vi "saveSequence.vi"(0 "object in":refnum<class "Hamamatsu.lvclass">, 2 "folder path":path, 5 "error in (no error)":errorcluster) -> (14 "object out":refnum<class "Hamamatsu.lvclass">, 16 "Timestamps":dbl[](array[numeric]), 17 "Filenames":path[](array[path]), 19 "error out":errorcluster)   [LabVIEW 2021, in "Hamamatsu.lvclass"]
uses:
  Hamamatsu.lvclass
  Hamamatsu.lvclass/Hamamatsu.ctl
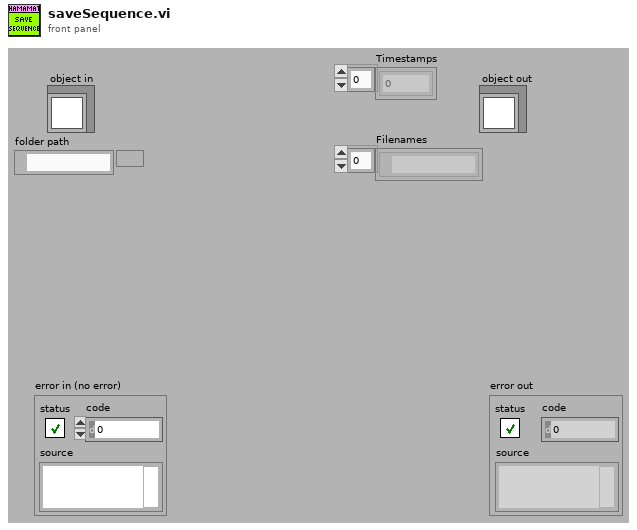
[diagram p1: front panel]
types:
  T1 = typedef "Image Type" = u32
  T2 = typedef "IMAQ Image.ctl" = refnum<image>
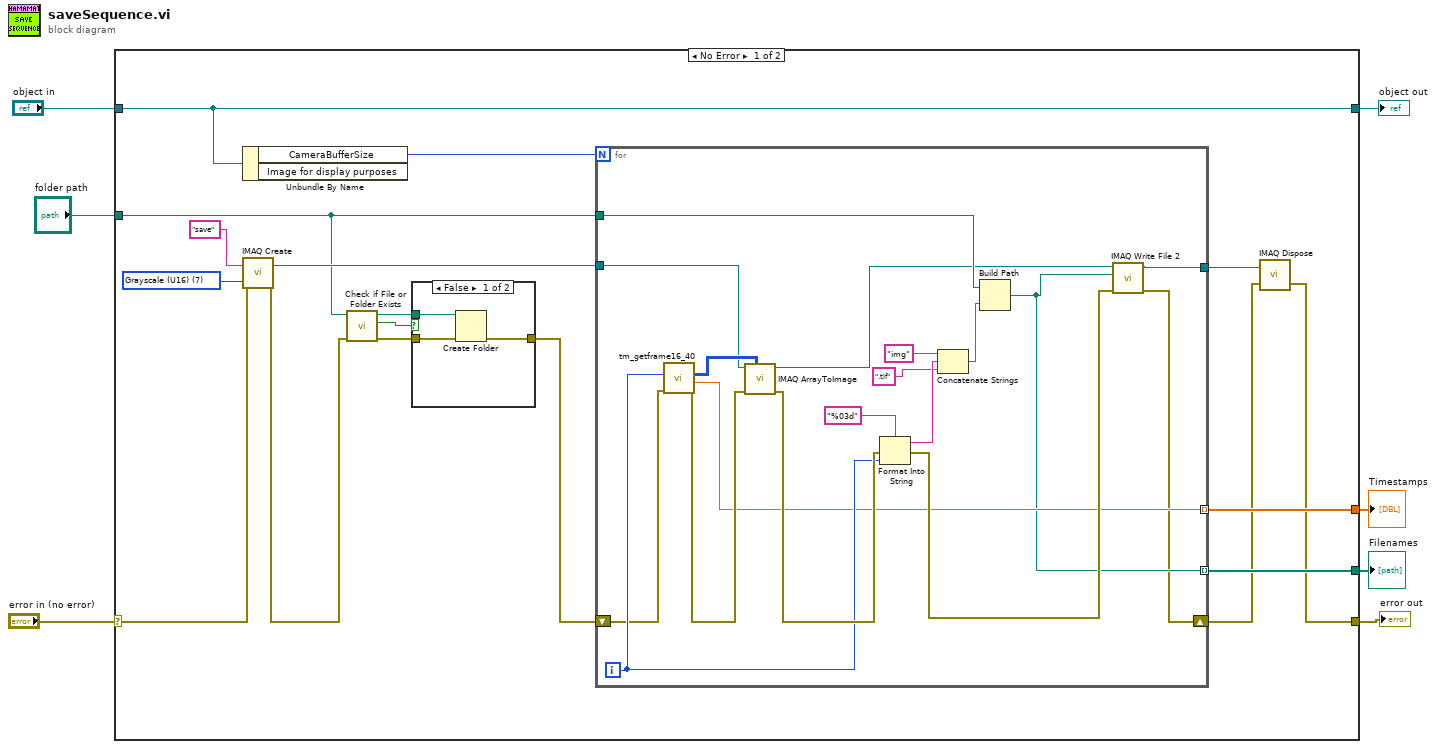
[diagram p0: block diagram]
diagram:
  n1 = case shown="No Error" "error in (no error)" {
    selector: "error in (no error)" -> [w19 w48]
    tunnel: [w14 w48] -> w6
    tunnel: [w24 w47] -> w4
    tunnel: "object in" -> [w24 w47]
    tunnel: "folder path" -> [w13 _]
    tunnel: [w18 _] -> w2
    tunnel: [w17 _] -> w1
    frame No Error {
      w20 = T1 7 items=["Grayscale (U8)", "Grayscale (I16)", "Grayscale (SGL)", "Complex (CSG)", "RGB (U32)", "HSL (U32)", "RGB (U64)", "Grayscale (U16)"] ("Image Type")
      n2 = Unbundle By Name(w24) -> ("CameraBufferSize"=w23:i32)  [unwired: 1 out]
      n3 = call "IMAQ Create"("Image Name"="save", "Image Type"=w20, "error in (no error)"=w19) -> ("New Image"=w21:T2, "error out"=w11:errorcluster)  [unwired: 2 in]
      n4 = call <vilib>:"Check if File or Folder Exists.vi"("error in (no error)"=w11, "path"=w13) -> ("error out"=w9:errorcluster, "file or folder exists?"=w10:bool, "dup path"=w12:path)  [unwired: 7 in]
      n5 = case shown="False" w10 {
        tunnel: w12 -> [w45 _]
        tunnel: w9 -> [w44 w46]
        tunnel: [w43 w46] -> w8
        frame False {
          n6 = Create Folder(path (use dialog)=w45, error in=w44) -> (error out=w43:errorcluster)  [unwired: 1 in, 2 out]
        }
        frame True {
        }
      }
      n7 = for {
        N: w23 -> [_]
        tunnel: w21 -> [w34]
        tunnel: w13 -> [w36]
        shift-right: [w25] -> w15
        shift-left: w8 -> [w31]
        tunnel: [w29] -> w18 mode=indexing
        tunnel: [w28] -> w17 mode=indexing
        tunnel: [w27] -> w16
        i -> [w32]
        n8 = call <userlib>:"tm_getframe16_40.vi"("error in (no error)"=w31, "Frame Index"=w32) -> ("error out"=w30:errorcluster, "Timestamp"=w29:dbl, "Data"=w35:u16[][])  [unwired: 6 in, 1 out]
        n9 = call "IMAQ ArrayToImage"("Image Pixels (U16)"=w35, "error in (no error)"=w30, "Image"=w34) -> ("error out"=w33:errorcluster, "Image Out"=w26:T2)  [unwired: 7 in]
        n10 = Format Into String(format string="%03d", error in=w33, w32) -> (resulting string=w40:string, error out=w38:errorcluster)  [unwired: 1 in]
        n11 = Concatenate Strings("img" ("string"), w40, ".tif" ("string")) -> (w39:string)
        n12 = Build Path(base path=w36, name or relative path=w39) -> (appended path=w28:path)
        n13 = call-poly "IMAQ Write File 2"("error in (no error)"=w38, "File Path"=w28, "Image"=w26) -> ("error out"=w25:errorcluster, "Image Out (duplicate)"=w27:T2)  [unwired: 7 in]
      }
      n14 = call "IMAQ Dispose"("Image"=w16, "error in (no error)"=w15) -> ("error out"=w14:errorcluster)  [unwired: 4 in]
    }
    frame Error {
    }
  }
  "error out" <- w6
  "object out" <- w4
  "Timestamps" <- w2
  "Filenames" <- w1
